vi "ProceListAction.vi"(9 "Btn_AutoRun":refnum<vi>, 11 "AutoRunFlg":refnum<vi>) -> (0 "error out":errorcluster, 2 "pause":bool)   [LabVIEW 2019]
uses:
  Function/Main UI/Glb/Main_UI Gb.vi
  MPC_VirbVision.lvclass
  LLB/Message/MsgShowAndLog.lvlib
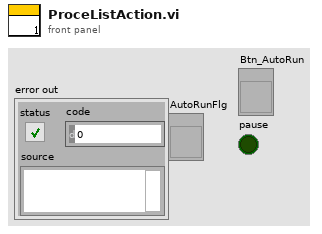
[diagram p1: front panel]
types:
  T1 = enum16{"Initial", "Write", "Read", "Save", "Load", "WrteAll"}
  T2 = cluster{"ProcessList":refnum<vi>, "Result Arr":refnum<vi>, "StopReceiveCmd":refnum<vi>}
  T3 = enum16{"initial", "write", "add", "delete", "Load", "Save", "Read", "ReadProjectName"}
  T4 = cluster{"ProjectName":string, "Parameter":string[][]}[]
  T5 = cluster{"ProjectName":string, "Parameter":string[][]}
  T6 = cluster{"ROI":string, "Numbers":i32, "Data":string[][]}[]
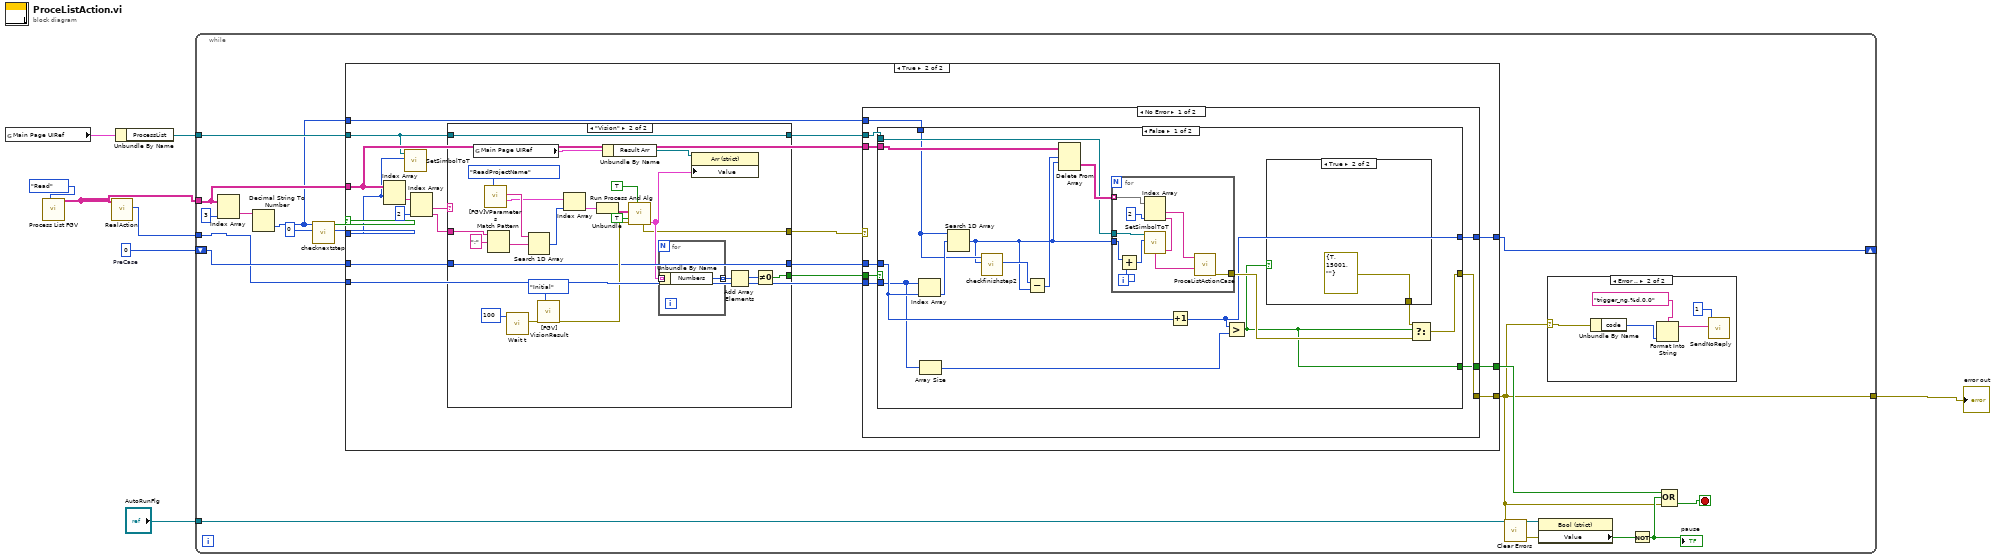
[diagram p0: block diagram]
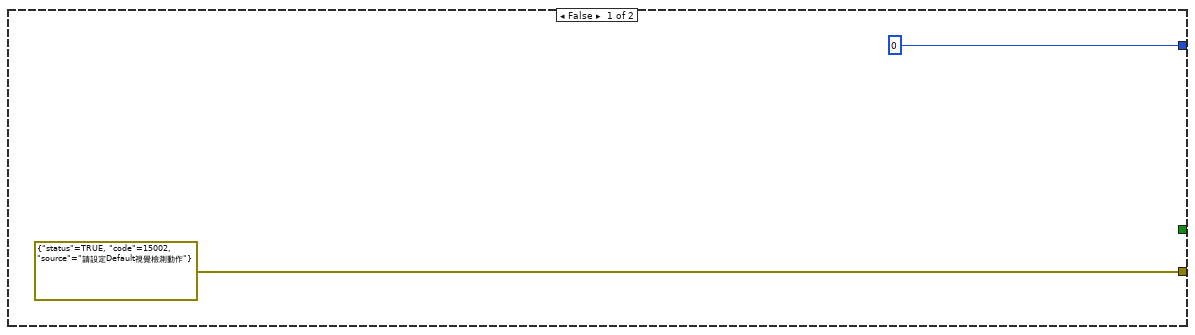
[diagram p3: hidden frame]
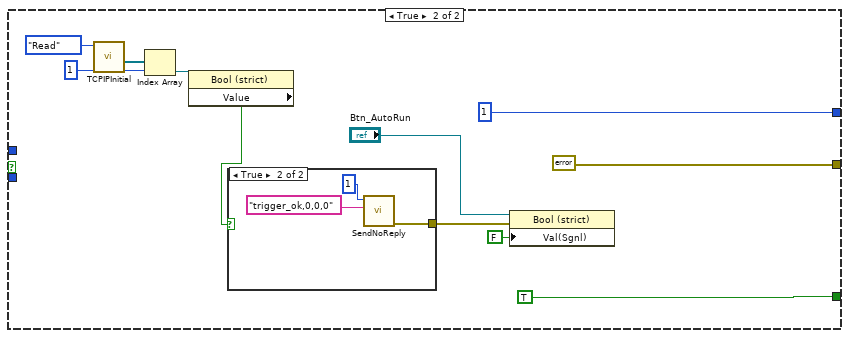
[diagram p5: hidden frame]
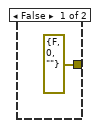
[diagram p6: hidden frame]
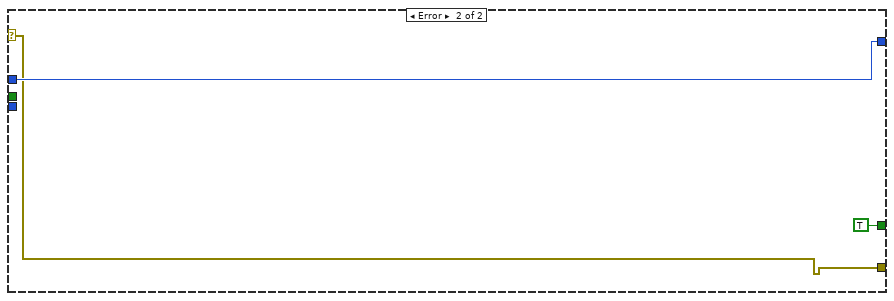
[diagram p7: hidden frame]
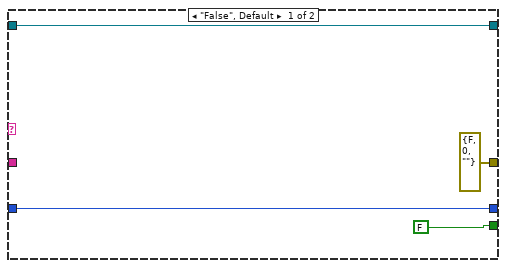
[diagram p8: hidden frame]
diagram:
  w8 = 0  # PreCase
  n1 = global read "Main_UI Gb.vi" "Main Page UIRef"() -> (w6:T2)
  n2 = call "Process List FGV.vi"("Action"=T1."Read") -> ("TableOut"=w1:string[][])  [unwired: 12 in, 2 out]
  n3 = call "RealAction.vi"("TableIn"=w1) -> ("Step"=w2:i32[])  [unwired: 9 in, 1 out]
  n4 = Unbundle By Name(w6) -> ("ProcessList"=w5:refnum<vi>)
  n5 = while {
    tunnel: [w10] -> w4
    shift-right: [w11] -> _
    shift-left: w8 -> [w21]
    tunnel: w1 -> [w23]
    tunnel: w5 -> [w17]
    tunnel: "AutoRunFlg" -> [w15]
    tunnel: w2 -> [w9]
    stop <- w20 stop-if-true
    n6 = Index Array(array=w23, index (col)=3 ("disabled index (col)")) -> (element=w25:string[])  [unwired: 1 in]
    n7 = Decimal String To Number(string=w25) -> (number=w13:i32[])  [unwired: 2 in, 1 out]
    n8 = call "checknextstep.vi"("Step"=0, "StepNumber"=w13) -> ("Index"=w22:i32, "ok"=w24:bool)  [unwired: 8 in]
    n9 = case shown="True" w24 {
      tunnel: [errorcluster {"status"=TRUE, "code"=15002, "source"="請設定Default視覺檢測動作"} ("error constant") w45] -> w10
      tunnel: w23 -> [_ w43]
      tunnel: w22 -> [_ w39]
      tunnel: w21 -> [_ w42]
      tunnel: [_ w41] -> w18
      tunnel: [0 w40] -> w11
      tunnel: w17 -> [_ w37]
      tunnel: w9 -> [_ w36]
      tunnel: w13 -> [_ w35]
      frame False {
      }
      frame True {
        n10 = Index Array(array=w43, index (row)=w39) -> (element=w50:string[])  [unwired: 1 in]
        n11 = call "SetSimbolToT.vi"("index"=w39, "ProcessList"=w37) -> ()  [unwired: 10 in]
        n12 = Index Array(array=w50, index #2=2 ("index")) -> (element #1=w49:string, element #2=w47:string)  [unwired: 1 in]
        n13 = case shown="\"Vision\"" w49 {
          tunnel: w47 -> [_ w131]
          tunnel: w42 -> [w106 w119]
          tunnel: [FALSE ("VisionOK") w117] -> w46
          tunnel: [w106 w119] -> w44
          tunnel: [w105 w118] -> w38
          tunnel: w37 -> [w105 w118]
          tunnel: [errorcluster {"status"=FALSE, "code"=0, "source"=""} ("error out") w108] -> w34
          frame "False", Default {
          }
          frame "Vision" {
            n14 = global read "Main_UI Gb.vi" "Main Page UIRef"() -> (w116:T2)
            n15 = call "[FGV]VParameters.vi"("Enum"=T3."ReadProjectName") -> ("Data"=w125:T4, "ProjectName"=w128:string[])  [unwired: 7 in, 2 out]
            n16 = Match Pattern(string=w131, regular expression=";") -> (after substring=w127:string)  [unwired: 1 in, 3 out]
            n17 = call "Wait t.vi"("wait(ms)"=u32 100) -> ("error out"=w111:errorcluster)  [unwired: 10 in]
            n18 = Search 1D Array(1D array=w128, element=w127) -> (index of element=w126:i32)  [unwired: 1 in]
            n19 = call "[FGV] VisionResult.vi"("Action"=T1."Initial", "error in"=w111) -> ("error out"=w120:errorcluster)  [unwired: 11 in, 2 out]
            n20 = Index Array(array=w125, index=w126) -> (element=w124:T5)
            n21 = Unbundle(w124) -> ("Parameter"=w123:string[][])  [unwired: 1 out]
            n22 = Unbundle By Name(w116) -> ("Result Arr"=w115:refnum<vi>)
            n23 = call "Run Process And Alg.vi"("Process"=TRUE, "error in (no error)"=w120, "CheckDist"=TRUE, "ROIList"=w123) -> ("Result Arr"=w114:T6, "error out"=w108:errorcluster)  [unwired: 3 in, 3 out]
            n24 = for {
              tunnel: w114 -> [w133] mode=indexing
              tunnel: [w132] -> w113 mode=indexing
              n25 = Unbundle By Name(w133) -> ("Numbers"=w132:i32)
            }
            n26 = property class="Arr (strict)"(reference=w115, "Value"=w114) -> ()  [unwired: 1 in, 2 out]
            n27 = Add Array Elements(numeric array=w113) -> (sum=w112:i32)
            n28 = Not Equal To 0?(x=w112) -> (x != 0?=w117:bool)
          }
        }
        n29 = case shown="No Error" w34 {
          selector: w34 -> [_ w101]
          tunnel: w46 -> [w59 _]
          tunnel: [w58 w101] -> w45
          tunnel: w44 -> [w57 w103]
          tunnel: w43 -> [w56 _]
          tunnel: [w55 TRUE] -> w41
          tunnel: [w54 w103] -> w40
          tunnel: w38 -> [w53 _]
          tunnel: w36 -> [w52 _]
          tunnel: w35 -> [w51 _]
          frame No Error {
            n30 = case shown="False" w59 {
              tunnel: [w71 errorcluster {"status"=FALSE, "code"=0, "source"="視覺結束"} ("error out")] -> w58
              tunnel: w57 -> [w68 _]
              tunnel: w56 -> [w75 _]
              tunnel: [w61 TRUE] -> w55
              tunnel: [w69 1] -> w54
              tunnel: w53 -> [w70 _]
              tunnel: w52 -> [w63 _]
              tunnel: w51 -> [w66 _]
              frame False {
                n31 = Index Array(array=w63, index=w68) -> (element=w67:i32)
                n32 = Array Size(array=w63) -> (size(s)=w62:i32)
                n33 = Search 1D Array(1D array=w66, element=w67) -> (index of element=w64:i32)  [unwired: 1 in]
                n34 = call "checkfinishstep2.vi"("Index"=w64, "StepNumber"=w66) -> ("Index"=w65:i32)  [unwired: 7 in, 2 out]
                n35 = Subtract(x=w65, y=w64) -> (x-y=w74:i32)
                n36 = Delete From Array(array=w75, length=w74, index (row)=w64) -> (deleted portion=w73:string[][])  [unwired: 1 in, 1 out]
                n37 = for {
                  tunnel: [w85] -> w72
                  tunnel: w73 -> [w84] mode=indexing
                  tunnel: w70 -> [w80]
                  tunnel: w64 -> [w77]
                  i -> [w79]
                  n38 = Add(x=w77, y=w79) -> (x+y=w78:i32)
                  n39 = Index Array(array=w84, index #2=2 ("index")) -> (element #1=w83:string, element #2=w82:string)  [unwired: 1 in]
                  n40 = call "SetSimbolToT.vi"("index"=w78, "ProcessList"=w80) -> ()  [unwired: 10 in]
                  n41 = call "ProceListActionCase.vi"("DataIn"=w82, "TypeIn"=w83) -> ("error out"=w85:errorcluster)  [unwired: 9 in]
                }
                n42 = Increment(x=w68) -> (x+1=w69:i32)
                n43 = Greater?(x=w69, y=w62) -> (0:w61:bool)
                n44 = case shown="True" w61 {
                  tunnel: [_ errorcluster {"status"=TRUE, "code"=15001, "source"=""} ("t")] -> w60
                  frame False {
                  }
                  frame True {
                  }
                }
                n45 = Select(t=w60, s=w61, f=w72) -> (s? t:f=w71:errorcluster)
              }
              frame True {
                n46 = call "TCPIPInitial.vi"("Enum"=enum16{"initial", "Read", "release"}."Read") -> ("Connect"=w89:refnum<vi>[])  [unwired: 7 in, 3 out]
                n47 = Index Array(array=w89, index=1) -> (element=w87:refnum<vi>)
                n48 = property class="Bool (strict)"(reference=w87) -> ("Value"=w86:bool)  [unwired: 1 in, 2 out]
                n49 = case shown="True" w86 {
                  tunnel: [errorcluster {"status"=FALSE, "code"=0, "source"=""} ("error out") w98] -> w92
                  frame False {
                  }
                  frame True {
                    n50 = call "SendNoReply.vi"("DataIn"="trigger_ok,0,0,0", "index"=1) -> ("error out"=w98:errorcluster)  [unwired: 9 in]
                  }
                }
                n51 = property class="Bool (strict)"(reference="Btn_AutoRun", error in=w92, "Val(Sgnl)"=FALSE ("Value")) -> ()  [unwired: 2 out]
              }
            }
          }
          frame Error {
          }
        }
      }
    }
    n52 = call <vilib>:"Clear Errors.vi"("error in (no error)"=w10) -> ("error out"=w14:errorcluster)  [unwired: 5 in, 1 out]
    n53 = property class="Bool (strict)"(reference=w15, error in=w14) -> ("Value"=w16:bool)  [unwired: 2 out]
    n54 = case shown="Error .." w10 {
      selector: w10 -> [_ w30]
      frame No Error {
      }
      frame Error {
        n55 = Unbundle By Name(w30) -> ("code"=w28:i32)
        n56 = Format Into String(format string="trigger_ng,%d,0,0" ("DataIn"), w28) -> (resulting string=w27:string)  [unwired: 2 in, 1 out]
        n57 = call "SendNoReply.vi"("DataIn"=w27, "index"=1) -> ()  [unwired: 9 in, 1 out]
      }
    }
    n58 = Not(x=w16) -> (.not. x?=w12:bool)
    "pause" <- w12
    n59 = Compound Arithmetic op=OR(w18, w12, w10) -> (w20:bool)
  }
  "error out" <- w4
